vi "parseCcdData.vi"(8 "error in (no error)":errorcluster, 11 "results-JSON string":string) -> (0 "error out":errorcluster, 3 "ccdData":T1[](array[typedef]))   [LabVIEW 2023, in "horiba.lvlib" / "CCD.lvclass"]
doc: "Helper VI to parse the ccd data to a LV 2D image array."
uses:
  CCD.lvclass
  acquisitionImageData.ctl
  imageAcqData.ctl
  ad48d047-c765-4916-affb-9fd3c0b9b783.vi
  c5adb225-65ff-4b52-aa76-4294a978254a.vi
  <vilib>/JDP Science/JSONtext/Next JSON Value.vi
  <vilib>/JDP Science/JSONtext/String Subset.vi
  <vilib>/JDP Science/JSONtext/Parsing/Advance past next JSON Value (inlined COPY).vi
  <vilib>/JDP Science/JSONtext/Parsing/Advance past whitespace.vi
  <vilib>/JDP Science/JSONtext/Parsing/Advance past String.vi
  <vilib>/JDP Science/JSONtext/Parsing/Advance past Number.vi
  <vilib>/JDP Science/JSONtext/Parsing/Advance past Line Ending.vi
  <vilib>/JDP Science/JSONtext/Parsing/Parse Full Path or Item Name.vi
  <vilib>/JDP Science/JSONtext/Parsing/Advance past Array.vi
  <vilib>/JDP Science/JSONtext/Parsing/Advance past Object.vi
  <vilib>/JDP Science/JSONtext/support/Error Cluster From Code.vi
  <vilib>/JDP Science/JSONtext/Offset/Find Item Locations by Path.vi
  <vilib>/JDP Science/JSONtext/JSON text to Variant.vi
  <vilib>/JDP Science/JSONtext/LVClass Serializer/JSONtext LVClass Serializer.lvclass
  <vilib>/JDP Science/JSONtext/JSONtext.lvlib
panel:
  # "Connector Pane"
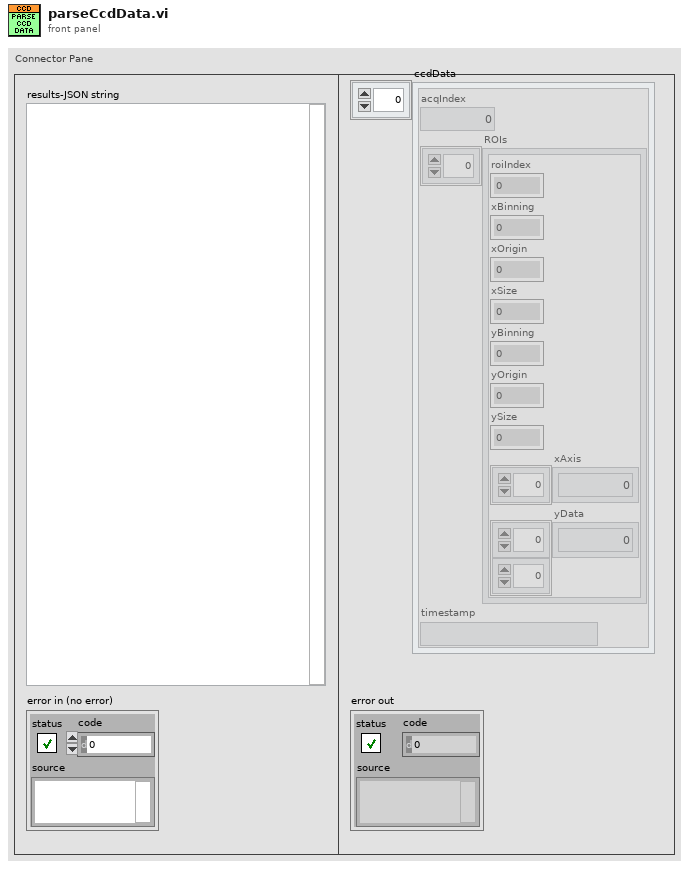
[diagram p1: front panel]
types:
  T1 = typedef "acquisitionImageData.ctl" = cluster{"acqIndex":i32, "ROIs":T2[], "timestamp":string}
  T2 = typedef "horiba.lvlib/CCD.lvclass/imageAcqData.ctl" = cluster{"roiIndex":i32, "xBinning":i32, "xOrigin":i32, "xSize":i32, "yBinning":i32, "yOrigin":i32, "ySize":i32, "xAxis":dbl[], "yData":dbl[][]}
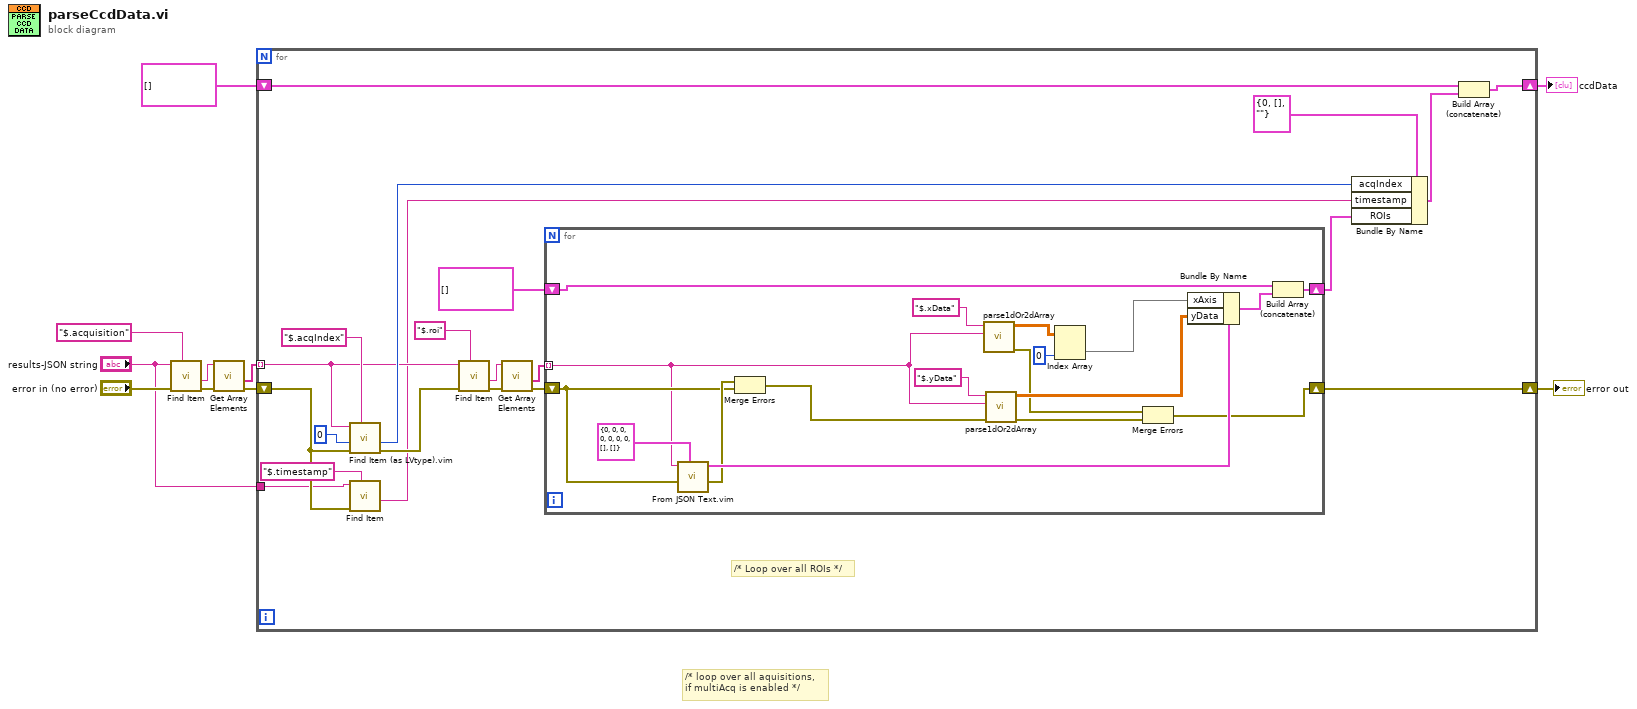
[diagram p0: block diagram]
diagram:
  # "/* loop over all aquisitions, \nif multiAcq is enabled */"
  n1 = call <vilib>:"Find Item.vi"("$Path or Item Name"="$.acquisition", "error in (no error)"="error in (no error)", "JSON"="results-JSON string") -> ("error out"=w7:errorcluster, "<JSON>"=w6:string)  [unwired: 5 in, 2 out]
  n2 = call <vilib>:"Get Array Elements.vi"("error in (no error)"=w7, "JSON"=w6) -> ("error out"=w10:errorcluster, "<JSON>"=w9:string[])  [unwired: 7 in, 1 out]
  n3 = for {
    tunnel: w9 -> [w16] mode=indexing
    shift-right: [w26] -> w5
    shift-left: w10 -> [w15]
    shift-right: [w17] -> w2
    shift-left: T1[] [] ("Array") -> [w20]
    tunnel: "results-JSON string" -> [w11]
    # "/* Loop over all ROIs */"
    n4 = call "Find Item (as LVtype).vim"("$Path or Item Name"="$.acqIndex", "error in (no error)"=w15, "Data Type and Default Value"=0, "JSON"=w16) -> ("error out"=w24:errorcluster, "Data"=w22:i32)  [unwired: 4 in, 2 out]
    n5 = call <vilib>:"Find Item.vi"("$Path or Item Name"="$.timestamp", "error in (no error)"=w15, "JSON"=w11) -> ("<JSON>"=w12:string)  [unwired: 5 in, 3 out]
    n6 = call <vilib>:"Find Item.vi"("$Path or Item Name"="$.roi", "error in (no error)"=w24, "JSON"=w16) -> ("error out"=w29:errorcluster, "<JSON>"=w30:string)  [unwired: 5 in, 2 out]
    n7 = call <vilib>:"Get Array Elements.vi"("error in (no error)"=w29, "JSON"=w30) -> ("error out"=w27:errorcluster, "<JSON>"=w28:string[])  [unwired: 7 in, 1 out]
    n8 = for {
      tunnel: w28 -> [w37] mode=indexing
      shift-right: [w34] -> w26
      shift-left: w27 -> [w46]
      shift-right: [w44] -> w13
      shift-left: T2[] [] -> [w43]
      n9 = call "From JSON Text.vim"("Data Type and Default Value"=T2 {"roiIndex"=0, "xBinning"=0, "xOrigin"=0, "xSize"=0, "yBinning"=0, "yOrigin"=0, "ySize"=0, "xAxis"=[], "yData"=[]} ("Data out"), "error in (no error)"=w46, "JSON"=w37) -> ("error out"=w47:errorcluster, "Data out"=w48:T2)  [unwired: 7 in]
      n10 = Merge Errors(w47, w46) -> (w42:errorcluster)
      n11 = call "parse1dOr2dArray.vi"("<JSON>"=w37, "$Path or Item Name"="$.xData") -> ("error out"=w33:errorcluster, "Data"=w36:dbl[][])  [unwired: 8 in]
      n12 = call "parse1dOr2dArray.vi"("error in (no error)"=w42, "<JSON>"=w37, "$Path or Item Name"="$.yData") -> ("error out"=w40:errorcluster, "Data"=w41:dbl[][])  [unwired: 7 in]
      n13 = Index Array(array=w36, index (col)=0 ("disabled index (col)")) -> (element=w35:dbl[])  [unwired: 1 in]
      n14 = Merge Errors(w33, w40) -> (w34:errorcluster)
      n15 = Bundle By Name(cluster=w48, "xAxis"=w35, "yData"=w41) -> (w45:T2)
      n16 = Build Array (concatenate)(w43, w45) -> (w44:T2[])
    }
    n17 = Bundle By Name(cluster=T1 {"acqIndex"=0, "ROIs"=[], "timestamp"=""} ("acquisition"), "acqIndex"=w22, "timestamp"=w12, "ROIs"=w13) -> (w18:T1)
    n18 = Build Array (concatenate)(w20, w18) -> (w17:T1[])
  }
  "error out" <- w5
  "ccdData" <- w2
